vi "VisionStuff1.22.2016.vi"() -> ()   [LabVIEW 2014]
uses:
  <vilib>/vision/Pattern Matching.llb/IMAQ GM Match Report.ctl
panel:
  out "Number of Matches (Geometric Matching 1)":i32
  out "Distance off Center of Picture in Pixels":dbl
  out "Calibrated Matches (Geometric Matching 1)":T1[](array[typedef]) {"Correlation Score" format="%.2f"; "Target Template Curve Score" format="%.2f"; "Template Target Curve Score" format="%.2f"; "Bounding Box"."y" format="%.2f"; "Bounding Box"."x" format="%.2f"; "Position"."y" format="%.2f"; "Position"."x" format="%.2f"; "Score" format="%.2f"; "Scale" format="%.2f"; "Angle" format="%.2f"; "Occlusion %" format="%.2f"}
  in  "Check for Logo":bool
  out "Matches (calibrated) (Color Location 1)":T2(array[cluster])
  in  "End Point":cluster{"X":i32, "Y":i32}
  in  "Start Point":cluster{"X":i32, "Y":i32}
  in  "Rectangle":T3
  in  "name":bool=TRUE
  out "name":string="roboRIO-2767.local"
  out "Camera Image":T4(plugin-control)
  out "Mbps":dbl=0.00015213946117274168 format="%#.1g"
  out "fps":dbl=0.08191171009807562 format="%#.1g"
  in  "Vision":u16(ring)=2 items=["Camera Off", "USB Camera SW", "USB Camera HW", "IP Camera"]
  # "USE ME------>"
  # "(doesn't do anything)"
  # "(ignore)"
  # "Ver 17"
  # "USE MINIMUM MATCH SCORE OF 625\nSTART ANGLE OF -7\nEND ANGLE OF 7\nNUMBER OF MATCHES 1"
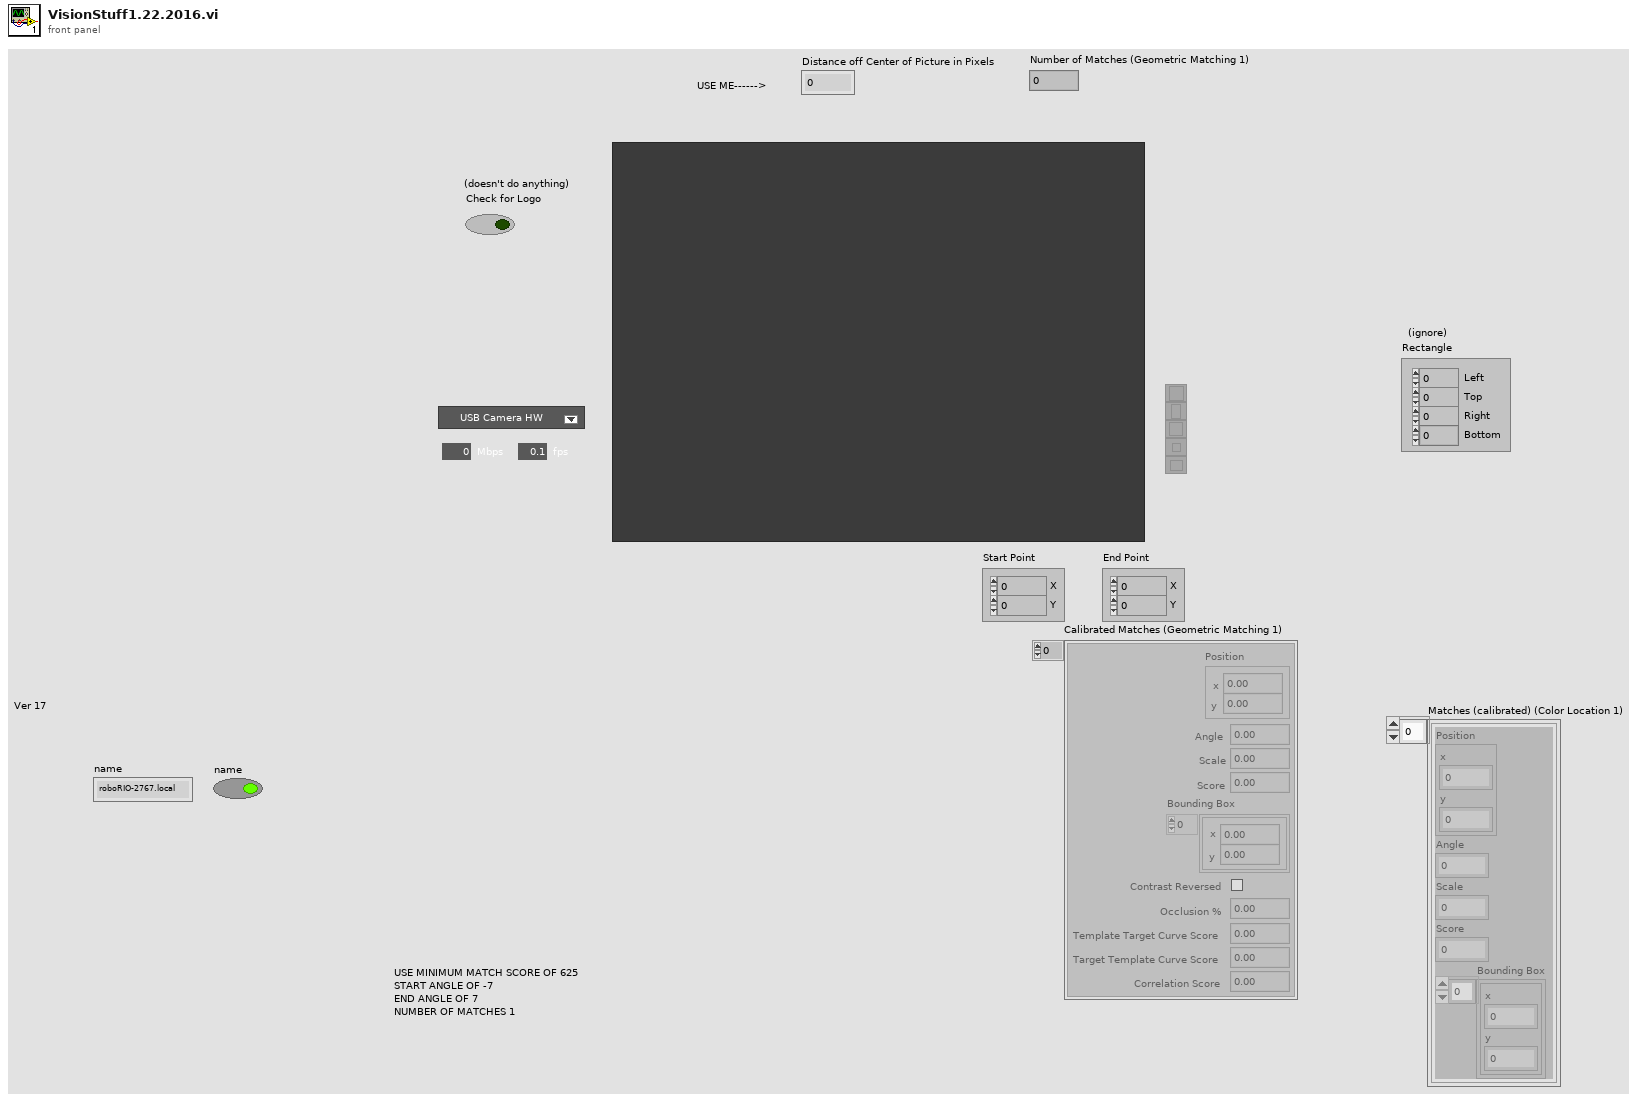
[diagram p1: front panel]
types:
  T1 = typedef "IMAQ GM Match Report.ctl" = cluster{"Position":cluster{"x":sgl, "y":sgl}, "Angle":sgl, "Scale":sgl, "Score":sgl, "Bounding Box":cluster{"x":sgl, "y":sgl}[], "Contrast Reversed":bool, "Occlusion %":sgl, "Template Target Curve Score":sgl, "Target Template Curve Score":sgl, "Correlation Score":sgl}
  T2 = cluster{"Position":cluster{"x":sgl, "y":sgl}, "Angle":sgl, "Scale":sgl, "Score":sgl, "Bounding Box":cluster{"x":sgl, "y":sgl}[]}[]
  T3 = cluster{"Left":i32, "Top":i32, "Right":i32, "Bottom":i32}
  T4 = typedef "IMAQ Image.ctl" = refnum<image>
  T5 = typedef "Image Type" = u32
  T6 = cluster{"Frame Rate":i32, "Compression":i32, "Size":u16}
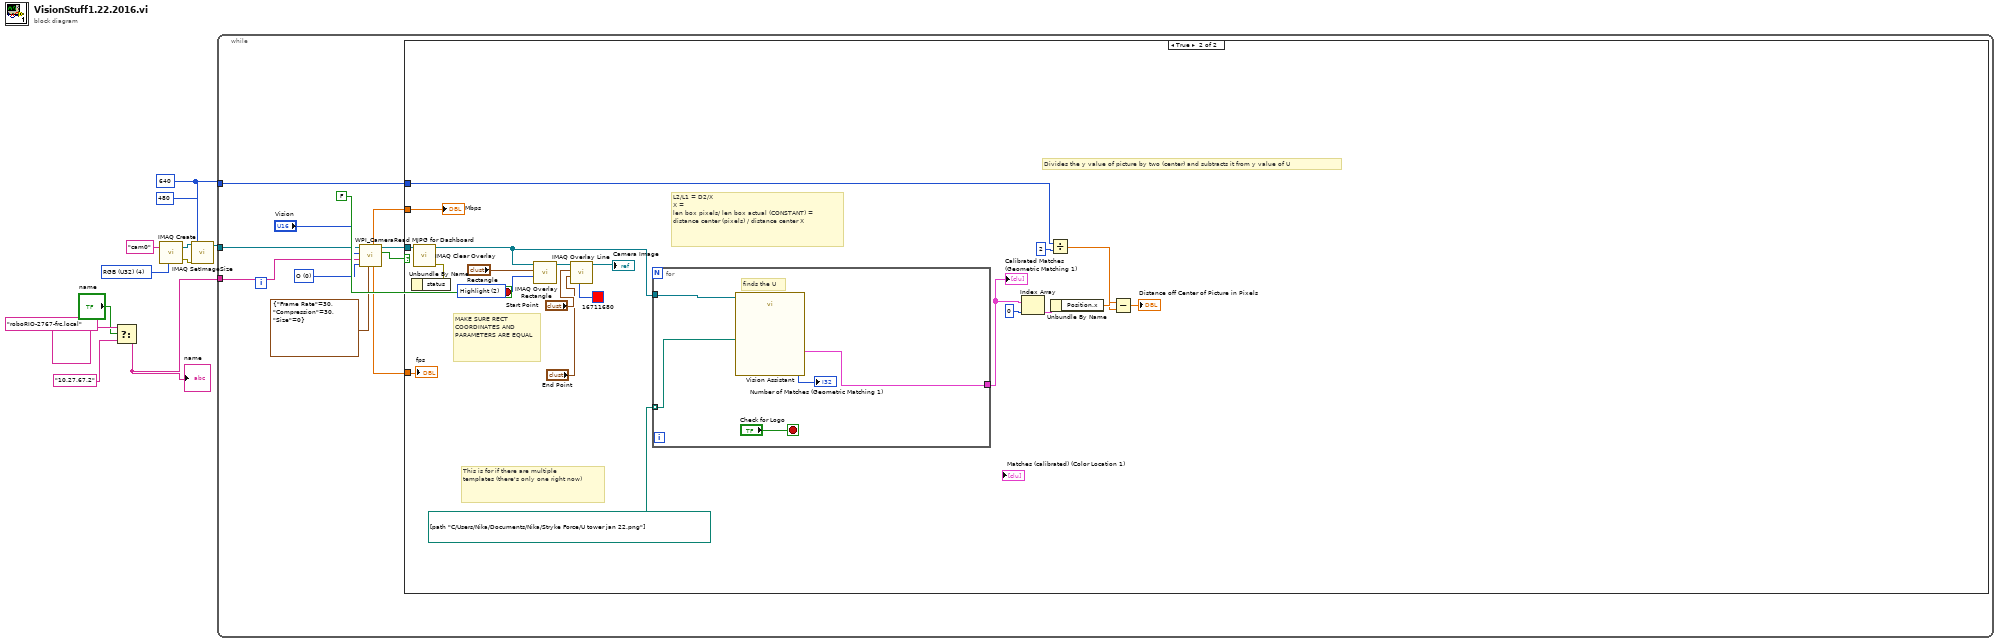
[diagram p0: block diagram]
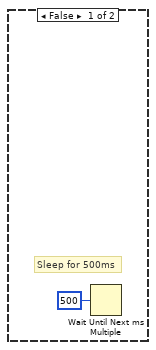
[diagram p2: hidden frame]
diagram:
  w1 = 640 ("X Resolution")
  w11 = T5 4 items=["Grayscale (U8)", "Grayscale (I16)", "Grayscale (SGL)", "Complex (CSG)", "RGB (U32)", "HSL (U32)", "RGB (U64)"] ("Image Type")
  n1 = Select(t="roboRIO-2767-frc.local" ("name"), s="name", f="10.27.67.2" ("name")) -> (s? t:f=w10:string)
  "name" <- w10
  n2 = call "IMAQ Create"("Image Name"="cam0", "Image Type"=w11) -> ("New Image"=w5:T4, "error out"=w4:errorcluster)  [unwired: 2 in, 1 out]
  n3 = call "IMAQ SetImageSize"("error in (no error)"=w4, "Y Resolution"=480, "X Resolution"=w1, "Image"=w5) -> ("Image Out"=w3:T4)  [unwired: 1 in, 1 out]
  n4 = while {
    tunnel: w3 -> [w14]
    tunnel: w10 -> [w15]
    tunnel: w1 -> [w12]
    stop <- FALSE stop-if-true
    w17 = u16 0 items=["O", "*", "Open Playback Panel"] ("Rec Mode")
    n5 = call <vilib>:"WPI_CameraRead MJPG for Dashboard.vi"("Camera Settings"=T6 {"Frame Rate"=30, "Compression"=30, "Size"=0}, "Rec Mode"=w17, "Camera IP"=w15, "Camera Mode"="Vision", "Refnum in"=w14) -> ("Active"=w20:bool, "Refnum out"=w21:T4, "FPS"=w19:dbl, "Bandwidth (Mbps)"=w18:dbl)  [unwired: 3 in]
    n6 = case shown="True" w20 {
      tunnel: w21 -> [_ w43]
      tunnel: w18 -> [_ w42]
      tunnel: w19 -> [_ w41]
      tunnel: w12 -> [_ w31]
      frame False {
        # "Sleep for 500ms"
        n7 = Wait Until Next ms Multiple(millisecond multiple=u32 500) -> ()  [unwired: 1 out]
      }
      frame True {
        w40 = u32 2 items=["Frame", "Fill", "Highlight"] ("Drawing Mode (Frame)")
        # "Divides the y value of picture by two (center) and subtracts it from y value of U"
        # "This is for if there are multiple templates (there's only one right now)"
        # "L2/L1 = D2/X\nX =  \nlen box pixels/ len box actual (CONSTANT) =\ndistance center (pixels) / distance center X"
        # "MAKE SURE RECT COORDINATES AND PARAMETERS ARE EQUAL"
        n8 = call "IMAQ Clear Overlay"("Image"=w43) -> ("error out"=w44:errorcluster, "Image Out"=w32:T4)  [unwired: 2 in, 7 out]
        n9 = Unbundle By Name(w44) -> ()  [unwired: 1 out]
        n10 = call "IMAQ Overlay Rectangle"("Drawing Mode (Frame)"=w40, "Rectangle"="Rectangle", "Image"=w32) -> ("Image Out"=w37:T4)  [unwired: 7 in, 1 out]
        n11 = call "IMAQ Overlay Line"("Color"=u32 16711680, "End Point"="End Point", "Start Point"="Start Point", "Image"=w37) -> ("Image Out"=→"Camera Image":T4)  [unwired: 6 in, 1 out]
        n12 = for {
          tunnel: w32 -> [w49]
          tunnel: path[] [path "C:/Users/Nika/Documents/Nika/Stryke Force/U tower jan 22.png"] -> [w46] mode=indexing
          tunnel: [w47] -> w29
          stop <- "Check for Logo" stop-if-true
          # "finds the U"
          n13 = call "Vision Assistant"("Image In"=w49, "Template File Path (Geometric Matching 1)"=w46) -> ("Number of Matches (Geometric Matching 1)"=→"Number of Matches (Geometric Matching 1)":i32, "Calibrated Matches (Geometric Matching 1)"=w47:T1[])  [unwired: 22 in, 2 out]
        }
        "Calibrated Matches (Geometric Matching 1)" <- w29
        n14 = Index Array(array=w29, index=0) -> (element=w27:T1)
        n15 = Divide(x=w31, y=2) -> (x/y=w24:dbl)
        n16 = Unbundle By Name(w27) -> ("Position.x"=w25:sgl)
        n17 = Subtract(x=w25, y=w24) -> (x-y=→"Distance off Center of Picture in Pixels":dbl)
        "Mbps" <- w42
        "fps" <- w41
      }
    }
  }
